vi "COMMinV2.vi"(0 "VISA resource name":refnum<visa-resource-name>) -> (1 "AtoDOut":i16, 2 "High Speed Count":i32)   [LabVIEW 2020]
uses:
  <vilib>/Instr/_visa.llb/VISA Set IO Buffer Mask.ctl
panel:
  in  "Mask":T1=16 items=["I/O Receive Buffer"=16, "I/O Transmit Buffer"=32, "I/O Receive and Transmit Buffer"=48]
  # "Data Aquisition Package - LabView and the NAIT Micro11 Board"
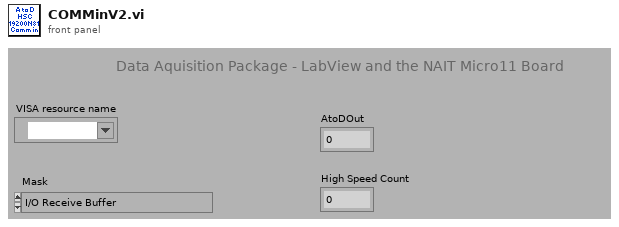
[diagram p1: front panel]
types:
  T1 = typedef "VISA Set IO Buffer Mask.ctl" = u16
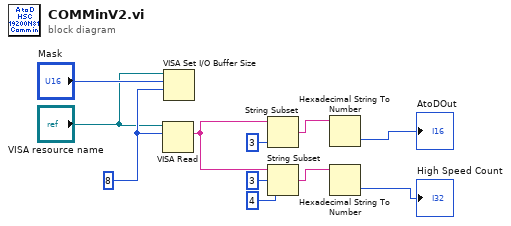
[diagram p0: block diagram]
diagram:
  w11 = 8
  n1 = VISA Read(VISA resource name="VISA resource name", byte count=w11) -> (read buffer=w8:string)  [unwired: 1 in, 3 out]
  n2 = VISA Set I/O Buffer Size(VISA resource name="VISA resource name", mask (16)="Mask", size (4096)=w11) -> ()  [unwired: 1 in, 2 out]
  n3 = String Subset(string=w8, length (rest)=3 ("length (rest)")) -> (substring=w4:string)  [unwired: 1 in]
  n4 = String Subset(string=w8, offset (0)=3, length (rest)=4 ("length (rest)")) -> (substring=w3:string)
  n5 = Hexadecimal String To Number(string=w4) -> (number=→"AtoDOut":u32)  [unwired: 2 in, 1 out]
  n6 = Hexadecimal String To Number(string=w3) -> (number=→"High Speed Count":u32)  [unwired: 2 in, 1 out]
